vi "YKMW100 Modbus Main.vi"(8 "error in (no error)":errorcluster, 11 "address":string="10.2.0.40") -> (0 "error out":errorcluster, 2 "MW Output":T1)   [LabVIEW 2023]
uses:
  Trunk/Hybrid Water Heater/Type Definitions/HEWH MW100 Data Cluster.ctl
  <vilib>/NI/Modbus Library/API/Wrapper/Create TCP Master.vi
  <vilib>/NI/Modbus Library/API/Master/Modbus Master.lvclass
  <vilib>/NI/Modbus Library/API/Wrapper/API Main.lvlib
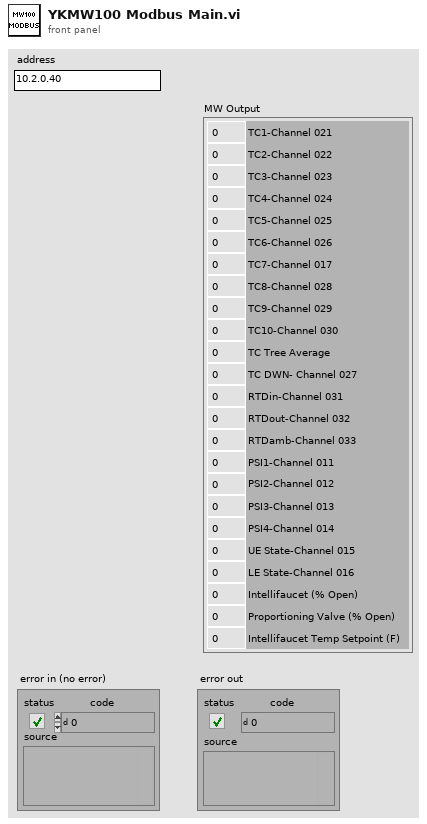
[diagram p1: front panel]
types:
  T1 = typedef "HEWH MW100 Data Cluster.ctl" = cluster{"TC1-Channel 021":dbl, "TC2-Channel 022":dbl, "TC3-Channel 023":dbl, "TC4-Channel 024":dbl, "TC5-Channel 025":dbl, "TC6-Channel 026":dbl, "TC7-Channel 017":dbl, "TC8-Channel 028":dbl, "TC9-Channel 029":dbl, "TC10-Channel 030":dbl, "TC Tree Average":dbl, "TC DWN- Channel 027":dbl, "RTDin-Channel 031":dbl, "RTDout-Channel 032":dbl, "RTDamb-Channel 033":dbl, "PSI1-Channel 011":dbl, "PSI2-Channel 012":dbl, "PSI3-Channel 013":dbl, "PSI4-Channel 014":dbl, "UE State-Channel 015":dbl, "LE State-Channel 016":dbl, "Intellifaucet (% Open)":dbl, "Proportioning Valve (% Open)":dbl, "Intellifaucet Temp Setpoint (F)":dbl}
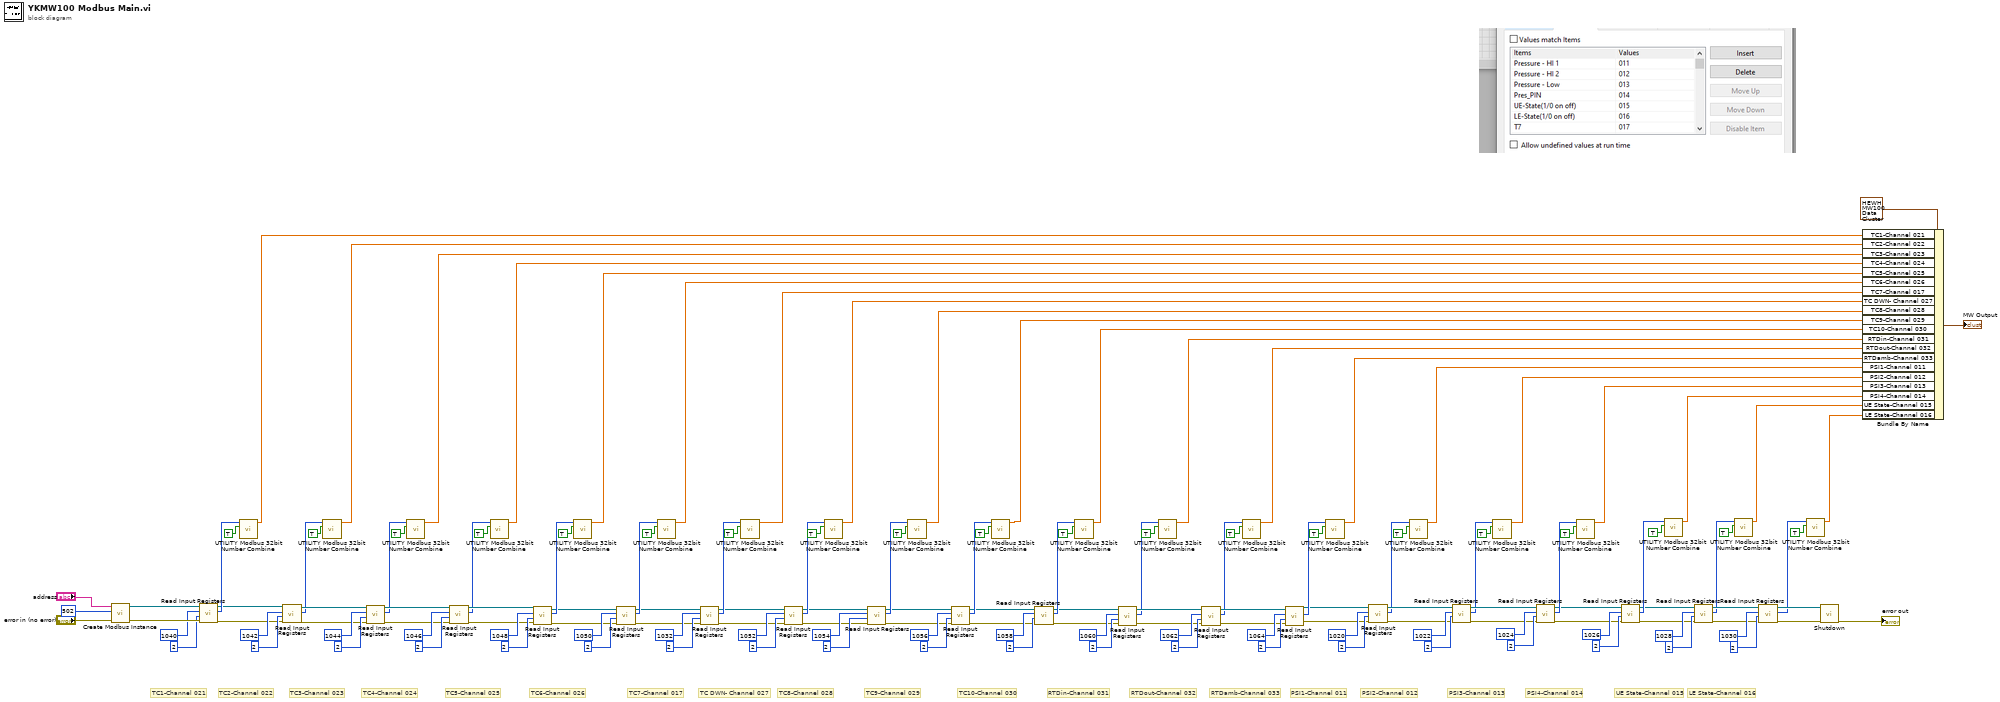
[diagram p0: block diagram]
diagram:
  # "LE State-Channel 016"
  # "UE State-Channel 015"
  # "PSI4-Channel 014"
  # "PSI3-Channel 013"
  # "PSI2-Channel 012"
  # "PSI1-Channel 011"
  # "RTDamb-Channel 033"
  # "RTDout-Channel 032"
  # "RTDin-Channel 031"
  # "TC10-Channel 030"
  # "TC9-Channel 029"
  # "TC8-Channel 028"
  # "TC DWN- Channel 027"
  # "TC7-Channel 017"
  # "TC6-Channel 026"
  # "TC5-Channel 025"
  # "TC4-Channel 024"
  # "TC3-Channel 023"
  # "TC2-Channel 022"
  # "TC1-Channel 021"
  n1 = call-poly <vilib>:"Create Modbus Instance.vi"("error in"="error in (no error)", "port (502)"=u16 502, "address"="address") -> ("error out"=w147:errorcluster, "TCP master instance"=w148:refnum<class "Modbus Master.lvclass">)  [unwired: 7 in]
  n2 = call-dynamic "Read Input Registers.vi"("error in"=w147, "number of inputs"=u16 2 ("Input Register number of inputs"), "starting address"=u16 1040 ("Input Register Starting address"), "Modbus master in"=w148) -> ("error out"=w135:errorcluster, "register values"=w142:u16[], "Modbus master out"=w136:refnum<class "Modbus Master.lvclass">)  [unwired: 5 in]
  n3 = call "UTILITY Modbus 32bit Number Combine.vi"("Swap Words"=TRUE, "Holding Registers"=w142) -> ("Data"=w41:sgl)  [unwired: 8 in, 1 out]
  n4 = call-dynamic "Read Input Registers.vi"("error in"=w135, "number of inputs"=u16 2 ("Input Register number of inputs"), "starting address"=u16 1042 ("Input Register Starting address"), "Modbus master in"=w136) -> ("error out"=w131:errorcluster, "register values"=w121:u16[], "Modbus master out"=w132:refnum<class "Modbus Master.lvclass">)  [unwired: 5 in]
  n5 = call "UTILITY Modbus 32bit Number Combine.vi"("Swap Words"=TRUE, "Holding Registers"=w121) -> ("Data"=w40:sgl)  [unwired: 8 in, 1 out]
  n6 = call-dynamic "Read Input Registers.vi"("error in"=w131, "number of inputs"=u16 2 ("Input Register number of inputs"), "starting address"=u16 1044 ("Input Register Starting address"), "Modbus master in"=w132) -> ("error out"=w127:errorcluster, "register values"=w119:u16[], "Modbus master out"=w128:refnum<class "Modbus Master.lvclass">)  [unwired: 5 in]
  n7 = call "UTILITY Modbus 32bit Number Combine.vi"("Swap Words"=TRUE, "Holding Registers"=w119) -> ("Data"=w39:sgl)  [unwired: 8 in, 1 out]
  n8 = call-dynamic "Read Input Registers.vi"("error in"=w127, "number of inputs"=u16 2 ("Input Register number of inputs"), "starting address"=u16 1046 ("Input Register Starting address"), "Modbus master in"=w128) -> ("error out"=w123:errorcluster, "register values"=w117:u16[], "Modbus master out"=w124:refnum<class "Modbus Master.lvclass">)  [unwired: 5 in]
  n9 = call "UTILITY Modbus 32bit Number Combine.vi"("Swap Words"=TRUE, "Holding Registers"=w117) -> ("Data"=w38:sgl)  [unwired: 8 in, 1 out]
  n10 = call-dynamic "Read Input Registers.vi"("error in"=w123, "number of inputs"=u16 2 ("Input Register number of inputs"), "starting address"=u16 1048 ("Input Register Starting address"), "Modbus master in"=w124) -> ("error out"=w112:errorcluster, "register values"=w115:u16[], "Modbus master out"=w111:refnum<class "Modbus Master.lvclass">)  [unwired: 5 in]
  n11 = call "UTILITY Modbus 32bit Number Combine.vi"("Swap Words"=TRUE, "Holding Registers"=w115) -> ("Data"=w37:sgl)  [unwired: 8 in, 1 out]
  n12 = call-dynamic "Read Input Registers.vi"("error in"=w112, "number of inputs"=u16 2 ("Input Register number of inputs"), "starting address"=u16 1050 ("Input Register Starting address"), "Modbus master in"=w111) -> ("error out"=w105:errorcluster, "register values"=w109:u16[], "Modbus master out"=w106:refnum<class "Modbus Master.lvclass">)  [unwired: 5 in]
  n13 = call "UTILITY Modbus 32bit Number Combine.vi"("Swap Words"=TRUE, "Holding Registers"=w109) -> ("Data"=w36:sgl)  [unwired: 8 in, 1 out]
  n14 = call-dynamic "Read Input Registers.vi"("error in"=w105, "number of inputs"=u16 2 ("Input Register number of inputs"), "starting address"=u16 1032 ("Input Register Starting address"), "Modbus master in"=w106) -> ("error out"=w49:errorcluster, "register values"=w103:u16[], "Modbus master out"=w50:refnum<class "Modbus Master.lvclass">)  [unwired: 5 in]
  n15 = call "UTILITY Modbus 32bit Number Combine.vi"("Swap Words"=TRUE, "Holding Registers"=w103) -> ("Data"=w35:sgl)  [unwired: 8 in, 1 out]
  n16 = call-dynamic "Read Input Registers.vi"("error in"=w49, "number of inputs"=u16 2 ("Input Register number of inputs"), "starting address"=u16 1052 ("Input Register Starting address"), "Modbus master in"=w50) -> ("error out"=w48:errorcluster, "register values"=w51:u16[], "Modbus master out"=w47:refnum<class "Modbus Master.lvclass">)  [unwired: 5 in]
  n17 = call "UTILITY Modbus 32bit Number Combine.vi"("Swap Words"=TRUE, "Holding Registers"=w51) -> ("Data"=w34:sgl)  [unwired: 8 in, 1 out]
  n18 = call-dynamic "Read Input Registers.vi"("error in"=w48, "number of inputs"=u16 2 ("Input Register number of inputs"), "starting address"=u16 1054 ("Input Register Starting address"), "Modbus master in"=w47) -> ("error out"=w58:errorcluster, "register values"=w59:u16[], "Modbus master out"=w46:refnum<class "Modbus Master.lvclass">)  [unwired: 5 in]
  n19 = call "UTILITY Modbus 32bit Number Combine.vi"("Swap Words"=TRUE, "Holding Registers"=w59) -> ("Data"=w33:sgl)  [unwired: 8 in, 1 out]
  n20 = call-dynamic "Read Input Registers.vi"("error in"=w58, "number of inputs"=u16 2 ("Input Register number of inputs"), "starting address"=u16 1056 ("Input Register Starting address"), "Modbus master in"=w46) -> ("error out"=w56:errorcluster, "register values"=w57:u16[], "Modbus master out"=w45:refnum<class "Modbus Master.lvclass">)  [unwired: 5 in]
  n21 = call "UTILITY Modbus 32bit Number Combine.vi"("Swap Words"=TRUE, "Holding Registers"=w57) -> ("Data"=w32:sgl)  [unwired: 8 in, 1 out]
  n22 = call-dynamic "Read Input Registers.vi"("error in"=w56, "number of inputs"=u16 2 ("Input Register number of inputs"), "starting address"=u16 1058 ("Input Register Starting address"), "Modbus master in"=w45) -> ("error out"=w43:errorcluster, "register values"=w55:u16[], "Modbus master out"=w44:refnum<class "Modbus Master.lvclass">)  [unwired: 5 in]
  n23 = call "UTILITY Modbus 32bit Number Combine.vi"("Swap Words"=TRUE, "Holding Registers"=w55) -> ("Data"=w31:sgl)  [unwired: 8 in, 1 out]
  n24 = call-dynamic "Read Input Registers.vi"("error in"=w43, "number of inputs"=u16 2 ("Input Register number of inputs"), "starting address"=u16 1060 ("Input Register Starting address"), "Modbus master in"=w44) -> ("error out"=w95:errorcluster, "register values"=w89:u16[], "Modbus master out"=w96:refnum<class "Modbus Master.lvclass">)  [unwired: 5 in]
  n25 = call "UTILITY Modbus 32bit Number Combine.vi"("Swap Words"=TRUE, "Holding Registers"=w89) -> ("Data"=w30:sgl)  [unwired: 8 in, 1 out]
  n26 = call-dynamic "Read Input Registers.vi"("error in"=w95, "number of inputs"=u16 2 ("Input Register number of inputs"), "starting address"=u16 1062 ("Input Register Starting address"), "Modbus master in"=w96) -> ("error out"=w94:errorcluster, "register values"=w88:u16[], "Modbus master out"=w93:refnum<class "Modbus Master.lvclass">)  [unwired: 5 in]
  n27 = call "UTILITY Modbus 32bit Number Combine.vi"("Swap Words"=TRUE, "Holding Registers"=w88) -> ("Data"=w29:sgl)  [unwired: 8 in, 1 out]
  n28 = call-dynamic "Read Input Registers.vi"("error in"=w94, "number of inputs"=u16 2 ("Input Register number of inputs"), "starting address"=u16 1064 ("Input Register Starting address"), "Modbus master in"=w93) -> ("error out"=w77:errorcluster, "register values"=w87:u16[], "Modbus master out"=w80:refnum<class "Modbus Master.lvclass">)  [unwired: 5 in]
  n29 = call "UTILITY Modbus 32bit Number Combine.vi"("Swap Words"=TRUE, "Holding Registers"=w87) -> ("Data"=w28:sgl)  [unwired: 8 in, 1 out]
  n30 = call-dynamic "Read Input Registers.vi"("error in"=w77, "number of inputs"=u16 2 ("Input Register number of inputs"), "starting address"=u16 1020 ("Input Register Starting address"), "Modbus master in"=w80) -> ("error out"=w76:errorcluster, "register values"=w71:u16[], "Modbus master out"=w79:refnum<class "Modbus Master.lvclass">)  [unwired: 5 in]
  n31 = call "UTILITY Modbus 32bit Number Combine.vi"("Swap Words"=TRUE, "Holding Registers"=w71) -> ("Data"=w27:sgl)  [unwired: 8 in, 1 out]
  n32 = call-dynamic "Read Input Registers.vi"("error in"=w76, "number of inputs"=u16 2 ("Input Register number of inputs"), "starting address"=u16 1022 ("Input Register Starting address"), "Modbus master in"=w79) -> ("error out"=w75:errorcluster, "register values"=w70:u16[], "Modbus master out"=w78:refnum<class "Modbus Master.lvclass">)  [unwired: 5 in]
  n33 = call "UTILITY Modbus 32bit Number Combine.vi"("Swap Words"=TRUE, "Holding Registers"=w70) -> ("Data"=w26:sgl)  [unwired: 8 in, 1 out]
  n34 = call-dynamic "Read Input Registers.vi"("error in"=w75, "number of inputs"=u16 2 ("Input Register number of inputs"), "starting address"=u16 1024 ("Input Register Starting address"), "Modbus master in"=w78) -> ("error out"=w22:errorcluster, "register values"=w69:u16[], "Modbus master out"=w21:refnum<class "Modbus Master.lvclass">)  [unwired: 5 in]
  n35 = call "UTILITY Modbus 32bit Number Combine.vi"("Swap Words"=TRUE, "Holding Registers"=w69) -> ("Data"=w25:sgl)  [unwired: 8 in, 1 out]
  n36 = call-dynamic "Read Input Registers.vi"("error in"=w22, "number of inputs"=u16 2 ("Input Register number of inputs"), "starting address"=u16 1026 ("Input Register Starting address"), "Modbus master in"=w21) -> ("error out"=w13:errorcluster, "register values"=w19:u16[], "Modbus master out"=w12:refnum<class "Modbus Master.lvclass">)  [unwired: 5 in]
  n37 = call "UTILITY Modbus 32bit Number Combine.vi"("Swap Words"=TRUE, "Holding Registers"=w19) -> ("Data"=w18:sgl)  [unwired: 8 in, 1 out]
  n38 = call-dynamic "Read Input Registers.vi"("error in"=w13, "number of inputs"=u16 2 ("Input Register number of inputs"), "starting address"=u16 1028 ("Input Register Starting address"), "Modbus master in"=w12) -> ("error out"=w10:errorcluster, "register values"=w8:u16[], "Modbus master out"=w11:refnum<class "Modbus Master.lvclass">)  [unwired: 5 in]
  n39 = call "UTILITY Modbus 32bit Number Combine.vi"("Swap Words"=TRUE, "Holding Registers"=w8) -> ("Data"=w5:sgl)  [unwired: 8 in, 1 out]
  n40 = call-dynamic "Read Input Registers.vi"("error in"=w10, "number of inputs"=u16 2 ("Input Register number of inputs"), "starting address"=u16 1030 ("Input Register Starting address"), "Modbus master in"=w11) -> ("error out"=w143:errorcluster, "register values"=w6:u16[], "Modbus master out"=w144:refnum<class "Modbus Master.lvclass">)  [unwired: 5 in]
  n41 = call "UTILITY Modbus 32bit Number Combine.vi"("Swap Words"=TRUE, "Holding Registers"=w6) -> ("Data"=w4:sgl)  [unwired: 8 in, 1 out]
  n42 = call-dynamic "Shutdown.vi"("error in"=w143, "Modbus master in"=w144) -> ("error out"=→"error out":errorcluster)  [unwired: 9 in]
  n43 = Bundle By Name(cluster=T1 {"TC1-Channel 021"=0.0, "TC2-Channel 022"=0.0, "TC3-Channel 023"=0.0, "TC4-Channel 024"=0.0, "TC5-Channel 025"=0.0, "TC6-Channel 026"=0.0, "TC7-Channel 017"=0.0, "TC8-Channel 028"=0.0, "TC9-Channel 029"=0.0, "TC10-Channel 030"=0.0, "TC Tree Average"=0.0, "TC DWN- Channel 027"=0.0, "RTDin-Channel 031"=0.0, "RTDout-Channel 032"=0.0, "RTDamb-Channel 033"=0.0, "PSI1-Channel 011"=0.0, "PSI2-Channel 012"=0.0, "PSI3-Channel 013"=0.0, "PSI4-Channel 014"=0.0, "UE State-Channel 015"=0.0, "LE State-Channel 016"=0.0, "Intellifaucet (% Open)"=0.0, "Proportioning Valve (% Open)"=0.0, "Intellifaucet Temp Setpoint (F)"=0.0} ("MW Input"), "TC1-Channel 021"=w41, "TC2-Channel 022"=w40, "TC3-Channel 023"=w39, "TC4-Channel 024"=w38, "TC5-Channel 025"=w37, "TC6-Channel 026"=w36, "TC7-Channel 017"=w35, "TC DWN- Channel 027"=w34, "TC8-Channel 028"=w33, "TC9-Channel 029"=w32, "TC10-Channel 030"=w31, "RTDin-Channel 031"=w30, "RTDout-Channel 032"=w29, "RTDamb-Channel 033"=w28, "PSI1-Channel 011"=w27, "PSI2-Channel 012"=w26, "PSI3-Channel 013"=w25, "PSI4-Channel 014"=w18, "UE State-Channel 015"=w5, "LE State-Channel 016"=w4) -> (→"MW Output":T1)
